vi "TDV_ReadJsonMetadata.vi"(8 "error in (no error)":errorcluster, 11 "JSON Source":path) -> (0 "error out":errorcluster, 3 "METADATA":T1)   [LabVIEW 2016]
uses:
  METADATA.ctl
  <vilib>/addons/_JKI.lib/Serialization/JSON/JKI JSON Serialization.lvlib
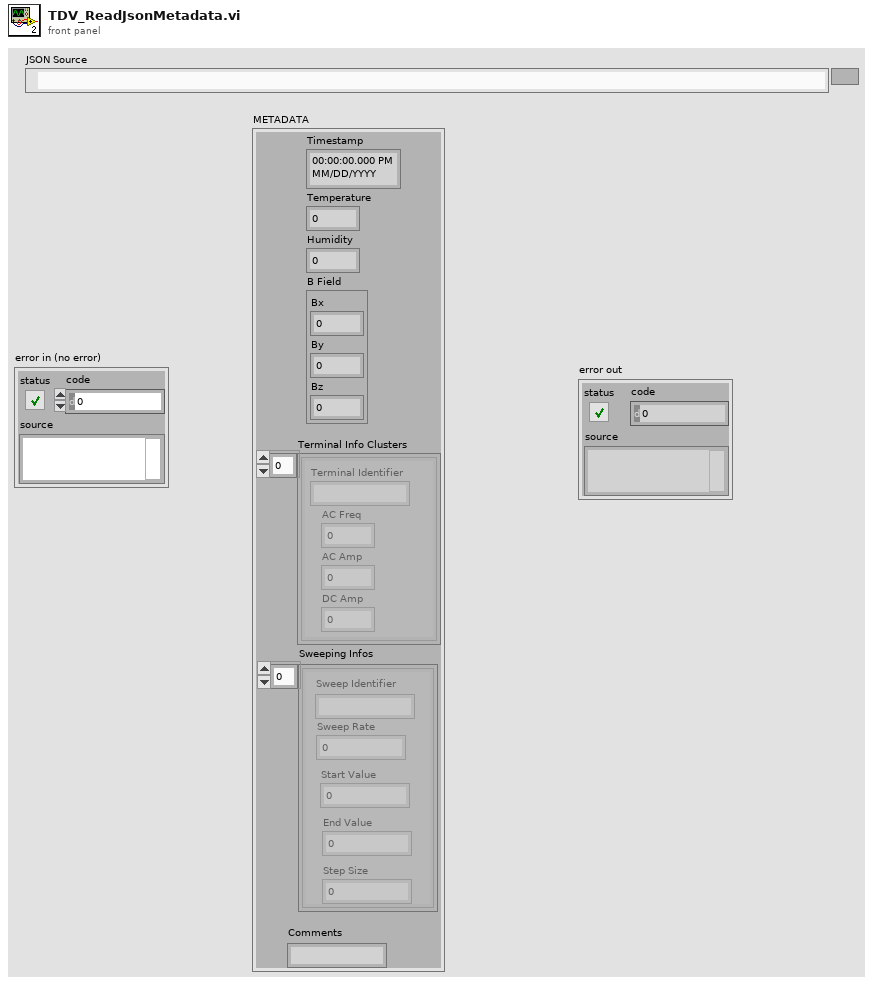
[diagram p1: front panel]
types:
  T1 = typedef "METADATA.ctl" = cluster{"Timestamp":timestamp, "Temperature":dbl, "Humidity":dbl, "B Field":cluster{"Bx":dbl, "By":dbl, "Bz":dbl}, "Terminal Info Clusters":cluster{"Terminal Identifier":string, "AC Freq":dbl, "AC Amp":dbl, "DC Amp":dbl}[], "Sweeping Infos":cluster{"Sweep Rate":dbl, "Sweep Identifier":string, "Start Value":dbl, "End Value":dbl, "Step Size":dbl}[], "Comments":string}
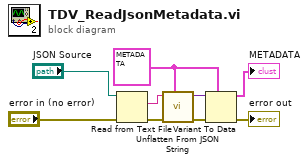
[diagram p0: block diagram]
diagram:
  w7 = T1 {"Timestamp"=timestamp(0 s since 1904-01-01), "Temperature"=0.0, "Humidity"=0.0, "B Field"={"Bx"=0.0, "By"=0.0, "Bz"=0.0}, "Terminal Info Clusters"=[], "Sweeping Infos"=[], "Comments"=""} ("Metadata Cluster")
  n1 = Read from Text File(file (use dialog)="JSON Source", error in="error in (no error)") -> (text=w5:string, error out=w3:errorcluster)  [unwired: 2 in, 2 out]
  n2 = call <vilib>:"Unflatten From JSON String.vi"("Type and Defaults"=w7, "error in (no error)"=w3, "JSON String"=w5) -> ("error out"=w2:errorcluster, "Variant"=w9:variant)  [unwired: 7 in]
  n3 = Variant To Data(error in=w2, type=w7, Variant=w9) -> (data=→"METADATA":T1, error out=→"error out":errorcluster)
